vi "RSZVB Get Trace Compression Point.vi"(8 "error in (no error)":errorcluster {"code" format="%.0x"}, 10 "Channel (Trace) (1)":i32=1, 11 "VISA session":refnum<visa-resource-name>) -> (0 "error out":errorcluster {"code" format="%.0x"}, 1 "Compression Point Out":dbl format="%^.3e", 2 "Compression Point In":dbl format="%^.3e", 3 "dup VISA session":refnum<visa-resource-name>)   [LabVIEW 2011]
doc: "This VI returns the x-dB compression point of an S-parameter or ratio measured in a power sweep. The compression value x is set via rszvb_SetTraceCompressionValue (CALCulate<Chn>:STATistics:NLINear:COMP:LEVel).\n\nNote(s):\n\n(1) An execution error message (error no. –200) is returned if no compression point is found.\n\nRemote-control command(s):\nCALCulate<Ch/Tr>:STATistics:NLINear:COMP:RESult?"
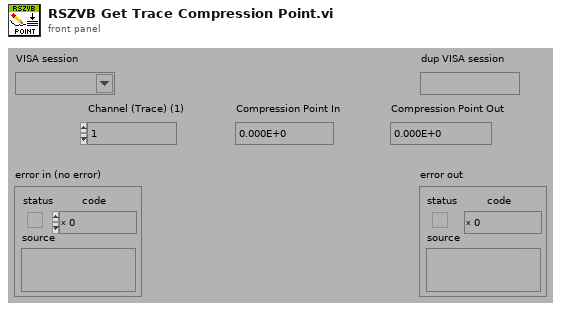
[diagram p1: front panel]
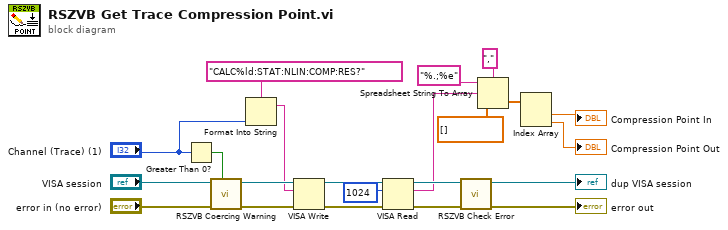
[diagram p0: block diagram]
diagram:
  n1 = Greater Than 0?(x="Channel (Trace) (1)") -> (x > 0?=w13:bool)
  n2 = call "RSZVB Coercing Warning.vi"("In Range?"=w13, "error in (no error)"="error in (no error)", "VISA session"="VISA session") -> ("error out"=w20:errorcluster, "dup VISA session"=w21:refnum<visa-resource-name>)  [unwired: 7 in]
  n3 = Format Into String(format string="CALC%ld:STAT:NLIN:COMP:RES?", "Channel (Trace) (1)") -> (resulting string=w19:string)  [unwired: 2 in, 1 out]
  n4 = VISA Write(VISA resource name=w21, write buffer=w19, error in (no error)=w20) -> (VISA resource name out=w16:refnum<visa-resource-name>, error out=w18:errorcluster)  [unwired: 1 out]
  n5 = VISA Read(VISA resource name=w16, byte count=u32 1024 ("byte count (0)"), error in (no error)=w18) -> (VISA resource name out=w15:refnum<visa-resource-name>, read buffer=w1:string, error out=w14:errorcluster)  [unwired: 1 out]
  n6 = call "RSZVB Check Error.vi"("error in (no error)"=w14, "VISA session"=w15) -> ("error out"=→"error out":errorcluster, "dup VISA session"=→"dup VISA session":refnum<visa-resource-name>)  [unwired: 8 in]
  n7 = Spreadsheet String To Array(delimiter (Tab)=",", format string="%.;%e", spreadsheet string=w1, array type (2D Dbl)=dbl[] []) -> (array=w2:dbl[])
  n8 = Index Array(array=w2) -> (element #1=→"Compression Point In":dbl, element #2=→"Compression Point Out":dbl)  [unwired: 2 in]
